vi "AndSpecification.vi"(10 "Specifications":refnum<class "IFilterSpecification.lvclass">[](array[class])) -> (3 "AndSpecification":refnum<class "AndSpecification.lvclass">)   [LabVIEW 2018, in "AndSpecification.lvclass"]
uses:
  AndSpecification.lvclass
  IFilterSpecification/IFilterSpecification.lvclass
  AndSpecification.lvclass/AndSpecification.ctl
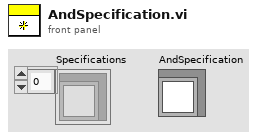
[diagram p1: front panel]
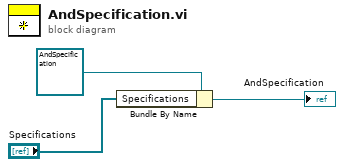
[diagram p0: block diagram]
diagram:
  n1 = Bundle By Name(cluster=refnum<class "AndSpecification.lvclass"> refnum ("AndSpecification.lvclass"), "Specifications"="Specifications") -> (→"AndSpecification":refnum<class "AndSpecification.lvclass">)
